vi "LVClass_Image save.vi"(0 "Image in":refnum<class "Image.lvclass">, 5 "Path (dialog if empty)":path, 7 "comments":string, 11 "error in (no error)":errorcluster) -> (4 "Image out":refnum<class "Image.lvclass">, 15 "error out":errorcluster)   [LabVIEW 2020, in "Image.lvclass"]
doc: "Load Image to file.\n\n--------------------------------------------------------------------------------\n\n<B>ImageIn </B> : Image object.\n<B>ImageOut </B> : Image object.\n<B>comments </B> : Comments to add.\n<B>image_file_path </B> : Absolute path to image file.\n<B>ErrorIn </B> : Error\n<B>ErrorOut </B> : Error\n\n--------------------------------------------------------------------------------"
uses:
  Image.lvclass
  Image.lvclass/Image.ctl
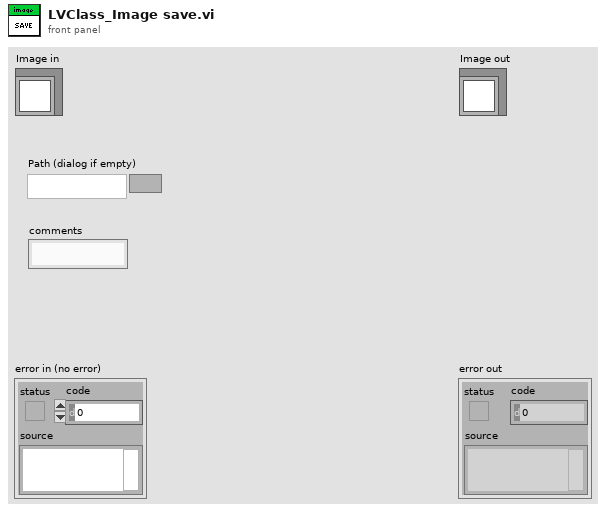
[diagram p1: front panel]
types:
  T1 = enum32{"existing file", "new file", "new or existing file", "existing dir", "new dir", "new or existing dir", "existing file (use LLBs)", "new file (use LLBs)", "new or existing file (use LLBs)", "new or existing file or directory (use LLBs)"}
  T2 = typedef "ClassID.ctl" = i64
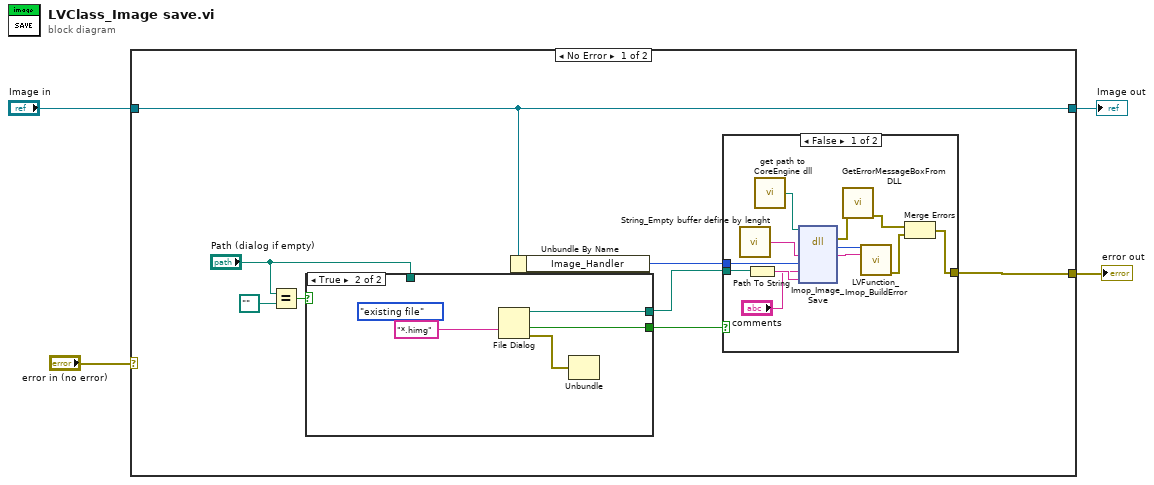
[diagram p0: block diagram]
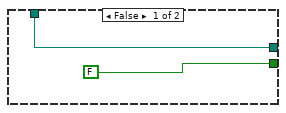
[diagram p3: hidden frame]
diagram:
  n1 = case shown="No Error" "error in (no error)" {
    selector: "error in (no error)" -> [_ w32]
    tunnel: [w7 w32] -> w3
    tunnel: [w6 w31] -> w1
    tunnel: "Image in" -> [w6 w31]
    frame No Error {
      n2 = Equal?(x="Path (dialog if empty)", y=path "") -> (x = y?=w12:bool)
      n3 = case shown="True" w12 {
        tunnel: [w26 w30] -> w8
        tunnel: "Path (dialog if empty)" -> [w26 _]
        tunnel: [FALSE ("cancelled") w29] -> w9
        frame False {
        }
        frame True {
          (unwired) T1."existing file" ("select mode (2)")
          n4 = File Dialog(6:"*.himg" ("pattern")) -> (0:w27:errorcluster, 1:w29:bool, 3:w30:path)  [unwired: 6 in, 1 out]
          n5 = Unbundle(w27) -> ()  [unwired: 3 out]
        }
      }
      n6 = Unbundle By Name(w6) -> ("Image_Handler"=w5:T2)
      n7 = case shown="False" w9 {
        tunnel: w8 -> [w22 _]
        tunnel: [w14 _] -> w7
        tunnel: w5 -> [w19 _]
        frame False {
          n8 = call "String_Empty buffer define by lenght.vi"() -> ("Empty buffer"=w24:string)  [unwired: 1 in]
          n9 = Path To String(path=w22) -> (string=w23:string)
          n10 = call "get path to CoreEngine dll.vi"() -> ("path to c_interface_vc100.dll"=w18:path)  [unwired: 12 in, 3 out]
          n11 = dll-call lib="D:/2_trunk/temp_core_engine/DLLs/ImopEngine4_vc100.dll" fn="Imop_Image_Save"(path in=w18, "message"=w24, "Image compat"=w19, "comments"="comments", "Path to image file"=w23) -> (error out=w17:errorcluster, "return type"=w21:i32, "message"=w20:string)  [unwired: 5 in, 1 out]
          n12 = call "GetErrorMessageBoxFromDLL.vi"("error IN"=w17) -> ("error OUT"=w16:errorcluster)  [unwired: 10 in]
          n13 = call "LVFunction_Imop_BuildError.vi"("code"=w21, "String to Prepend to source (\"\")"=w20) -> ("error out"=w15:errorcluster)  [unwired: 13 in]
          n14 = Merge Errors(w16, w15) -> (w14:errorcluster)
        }
        frame True {
        }
      }
    }
    frame Error {
    }
  }
  "error out" <- w3
  "Image out" <- w1
